vi "Add Label.vi"(8 "error in":errorcluster, 10 "label configuration":T1 {"sdi" items=["All", "Item00", "Item01", "Item10", "Item11"]}, 11 "channel in":refnum<k24>) -> (0 "error out":errorcluster, 2 "new label":refnum<k24>, 3 "channel out":refnum<k24>)   [LabVIEW 2020, in "Ballard_Parameter_ni.lvlib"]
uses:
  C:/Users/Administrator/Desktop/GIT/Ballard-Arinc-429-XML-Generator/Source/Assemblies/Ballard_Parameter_ni/bin/Debug/Parameters_Arinc429_XML_Tools.dll
  Assemblies/Ballard_Parameter_ni/bin/Debug/Parameters_Arinc429_XML_Tools.dll
  Ballard_Parameter_ni.lvlib
  _tyedefs/label_type.ctl
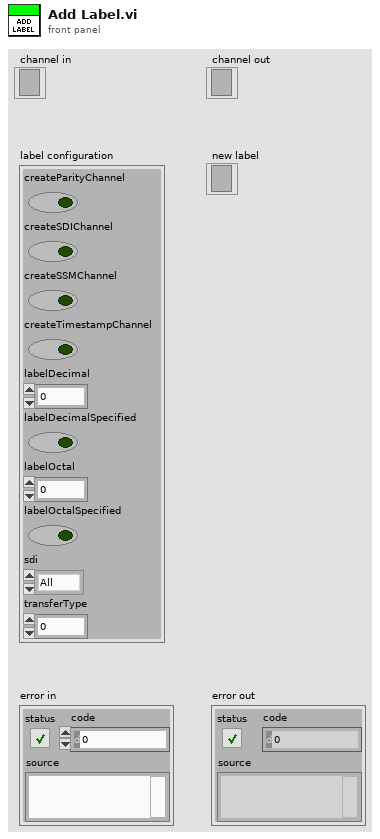
[diagram p1: front panel]
types:
  T1 = typedef "label_type.ctl" = cluster{"createParityChannel":bool, "createSDIChannel":bool, "createSSMChannel":bool, "createTimestampChannel":bool, "labelDecimal":i32, "labelDecimalSpecified":bool, "labelOctal":i32, "labelOctalSpecified":bool, "sdi":i32, "transferType":i32}
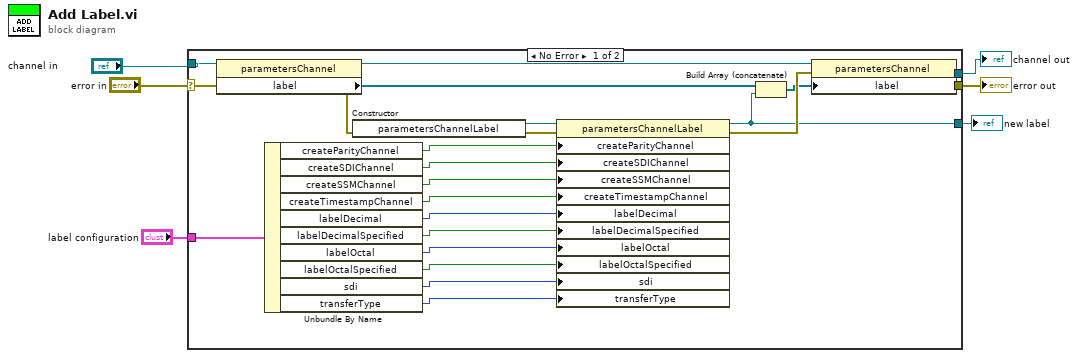
[diagram p0: block diagram]
diagram:
  n1 = case shown="No Error" "error in" {
    selector: "error in" -> [w28 w30]
    tunnel: [w24 w31] -> w6
    tunnel: [w23 w30] -> w5
    tunnel: "channel in" -> [w29 w31]
    tunnel: [w8 _] -> w1
    tunnel: "label configuration" -> [w19 _]
    frame No Error {
      n2 = property class="parametersChannel"(reference=w29, error in=w28) -> (reference out=w25:refnum<k24>, error out=w26:errorcluster, "label"=w27:refnum<k24>[])
      n3 = Unbundle By Name(w19) -> ("createParityChannel"=w18:bool, "createSDIChannel"=w17:bool, "createSSMChannel"=w16:bool, "createTimestampChannel"=w15:bool, "labelDecimal"=w14:i32, "labelDecimalSpecified"=w13:bool, "labelOctal"=w12:i32, "labelOctalSpecified"=w11:bool, "sdi"=w10:i32, "transferType"=w9:i32)
      n4 = constructor class="parametersChannelLabel"(error in=w26) -> (reference out=w22:refnum<k24>, error out=w21:errorcluster)  [unwired: 2 in, 1 out]
      n5 = property class="parametersChannelLabel"(reference=w22, error in=w21, "createParityChannel"=w18, "createSDIChannel"=w17, "createSSMChannel"=w16, "createTimestampChannel"=w15, "labelDecimal"=w14, "labelDecimalSpecified"=w13, "labelOctal"=w12, "labelOctalSpecified"=w11, "sdi"=w10, "transferType"=w9) -> (reference out=w8:refnum<k24>, error out=w20:errorcluster)
      n6 = Build Array (concatenate)(w27, w8) -> (w7:refnum<k24>[])
      n7 = property class="parametersChannel"(reference=w25, error in=w20, "label"=w7) -> (reference out=w24:refnum<k24>, error out=w23:errorcluster)
    }
    frame Error {
    }
  }
  "channel out" <- w6
  "error out" <- w5
  "new label" <- w1
